vi "test library.vi"() -> ()   [LabVIEW 2019, in "infolib.lvlib"]
uses:
  infolib.lvlib
  I64.vi
  String.vi
  Time Stamp.vi
  Boolean.vi
  1D CXT.vi
  2D EXT.vi
panel:
  in  "filename to write":path=path "c:/a"
  in  "2D array":dbl[][](array[numeric])=[[1.0, 3.0], [2.0, 4.0]]
  in  "1D array":dbl[](array[numeric])=[1.0, 2.0]
  in  "time stamp":timestamp
  out "all fields test":string
  in  "Numeric":i64=1
  out "section do exist, section is set":string
  out "section do not exist, section is set":string
  out "section do exist, section and subsection is not set":string
  out "section do not exist, section and subsection is not set":string
  out "section do exist, section and subsection is set":string
  out "section do not exist, section and subsection is set":string
  # "because labview internally uses newlines as lf (i.e. string control generates always\nlf independentally on local settings), set in project properties-conditional disables symbols-EOL as lf \nfor testing purposes."
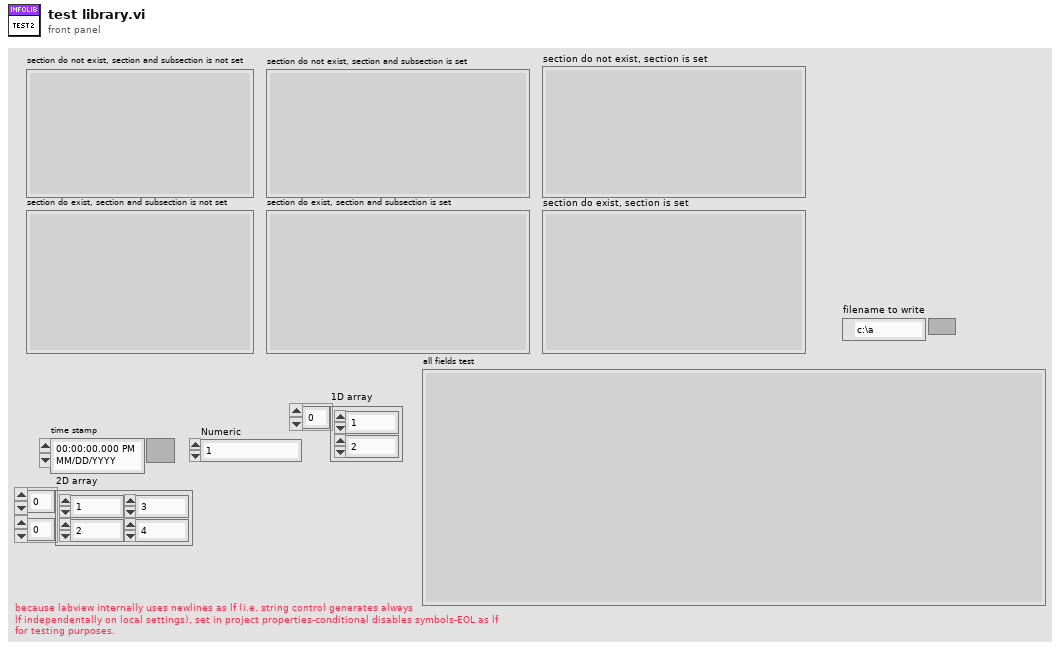
[diagram p1: front panel]
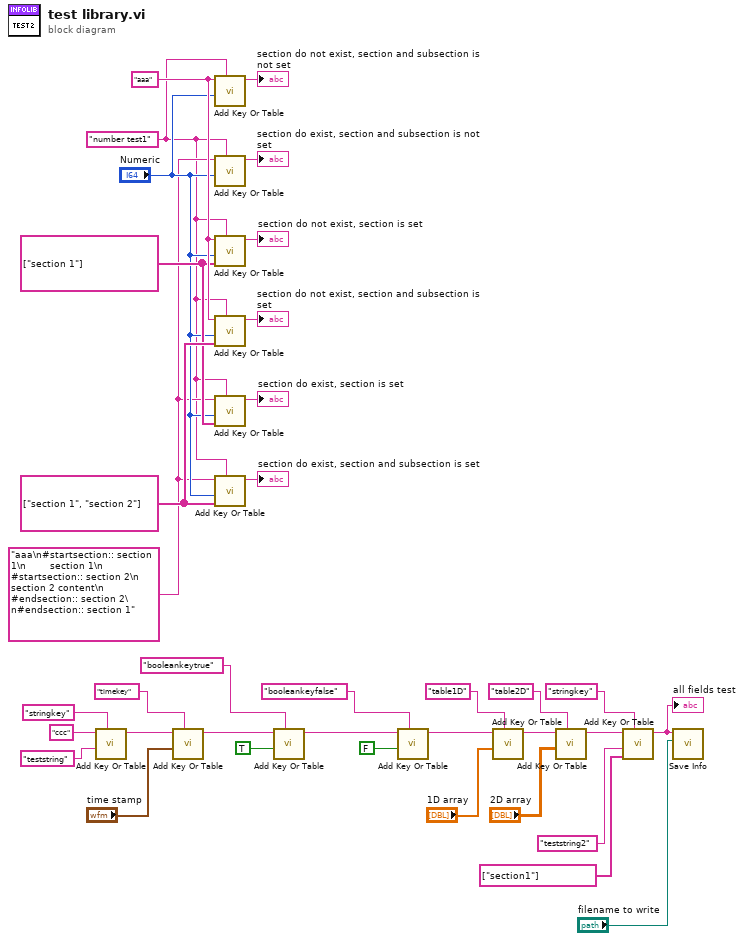
[diagram p0: block diagram]
diagram:
  w28 = string[] ["section 1"] ("sections")
  w31 = string[] ["section 1", "section 2"] ("sections")
  w8 = "number test1" ("key description")
  w30 = "aaa" ("info data")
  w25 = "aaa\n#startsection:: section 1\n        section 1\n        #startsection:: section 2\n                section 2 content\n        #endsection:: section 2\n#endsection:: section 1" ("info data")
  n1 = call-poly "Add Key Or Table.vi"("key description"="stringkey", "string"="teststring", "info data"="ccc") -> ("info data out"=w23:string)  [unwired: 7 in, 1 out]
  n2 = call-poly "Add Key Or Table.vi"("key description"="timekey", "time stamp"="time stamp", "info data"=w23) -> ("info data out"=w21:string)  [unwired: 7 in, 1 out]
  n3 = call-poly "Add Key Or Table.vi"("key description"=w8, "numeric"="Numeric", "info data"=w30) -> ("info data out"=→"section do not exist, section and subsection is not set":string)  [unwired: 7 in, 1 out]
  n4 = call-poly "Add Key Or Table.vi"("key description"=w8, "numeric"="Numeric", "info data"=w25) -> ("info data out"=→"section do exist, section and subsection is not set":string)  [unwired: 7 in, 1 out]
  n5 = call-poly "Add Key Or Table.vi"("key description"=w8, "sections"=w28, "numeric"="Numeric", "info data"=w30) -> ("info data out"=→"section do not exist, section is set":string)  [unwired: 6 in, 1 out]
  n6 = call-poly "Add Key Or Table.vi"("key description"=w8, "sections"=w31, "numeric"="Numeric", "info data"=w30) -> ("info data out"=→"section do not exist, section and subsection is set":string)  [unwired: 6 in, 1 out]
  n7 = call-poly "Add Key Or Table.vi"("key description"=w8, "sections"=w28, "numeric"="Numeric", "info data"=w25) -> ("info data out"=→"section do exist, section is set":string)  [unwired: 6 in, 1 out]
  n8 = call-poly "Add Key Or Table.vi"("key description"=w8, "sections"=w31, "numeric"="Numeric", "info data"=w25) -> ("info data out"=→"section do exist, section and subsection is set":string)  [unwired: 6 in, 1 out]
  n9 = call-poly "Add Key Or Table.vi"("key description"="booleankeytrue", "boolean"=TRUE ("Boolean"), "info data"=w21) -> ("info data out"=w18:string)  [unwired: 7 in, 1 out]
  n10 = call-poly "Add Key Or Table.vi"("key description"="booleankeyfalse", "boolean"=FALSE ("Boolean 2"), "info data"=w18) -> ("info data out"=w16:string)  [unwired: 7 in, 1 out]
  n11 = call-poly "Add Key Or Table.vi"("key description"="table1D", "numeric"="1D array", "info data"=w16) -> ("info data out"=w15:string)  [unwired: 7 in, 1 out]
  n12 = call-poly "Add Key Or Table.vi"("key description"="table2D", "numeric"="2D array", "info data"=w15) -> ("info data out"=w12:string)  [unwired: 7 in, 1 out]
  n13 = call-poly "Add Key Or Table.vi"("key description"="stringkey", "sections"=string[] ["section1"], "string"="teststring2", "info data"=w12) -> ("info data out"=w9:string)  [unwired: 6 in, 1 out]
  "all fields test" <- w9
  n14 = call "Save Info.vi"("filename"="filename to write", "info data"=w9) -> ()  [unwired: 9 in, 1 out]
